vi "Dpc Get Reg Set.vi"(0 "hif":u32, 1 "perc":i32, 5 "rgbAddr":string, 7 "rgbData":string, 9 "cbData":i32, 11 "error in (no error)":errorcluster, 12 "ptrid":u16) -> (3 "perc out":i32, 4 "hif out":u32, 6 "rgbAddr out":string, 8 "rgbData out":string, 10 "function return":i32, 14 "ptrid out":u16, 15 "error out":errorcluster)   [LabVIEW 2011, in "LVH-Adept.lvlib" / "DPCUTIL.lvlib"]
doc: "DPCAPI BOOL DpcGetRegSet(HANDLE hif, BYTE * rgbAddr, BYTE * rgbData, INT32 cbData, ERC * perc, TRID * ptrid);"
uses:
  DPCUTIL.lvlib
  Resources/dpcutil.dll
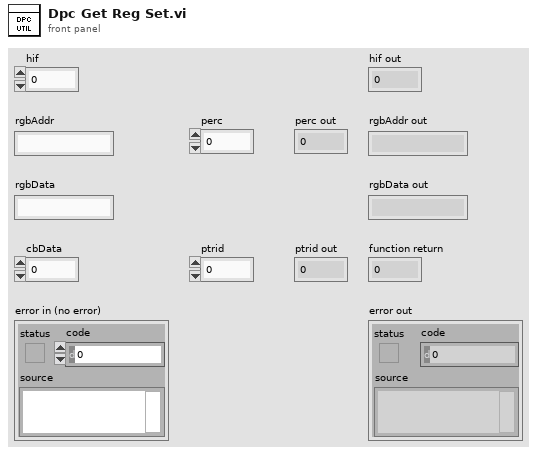
[diagram p1: front panel]
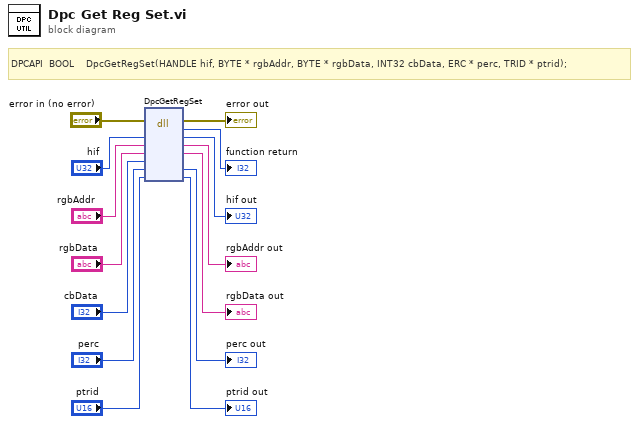
[diagram p0: block diagram]
diagram:
  # "DPCAPI  BOOL    DpcGetRegSet(HANDLE hif, BYTE * rgbAddr, BYTE * rgbData, INT32 cbData, ERC * perc, TRID * ptrid);"
  n1 = dll-call lib="C:/github/labviewhacker/LVH-Adept/LabVIEW/vi.lib/LabVIEW Hacker/Adept/Private/Resources/dpcutil.*" fn="DpcGetRegSet"(error in="error in (no error)", "hif"="hif", "rgbAddr"="rgbAddr", "rgbData"="rgbData", "cbData"="cbData", "perc"="perc", "ptrid"="ptrid") -> (error out=→"error out":errorcluster, →"function return":i32, "hif"=→"hif out":u32, "rgbAddr"=→"rgbAddr out":string, "rgbData"=→"rgbData out":string, "perc"=→"perc out":i32, "ptrid"=→"ptrid out":u16)  [unwired: 3 in, 1 out]
